vi "A2ii.vi"() -> ()   [LabVIEW 2020]
panel:
  out "Table":string[][](table)
  in  "stop":bool
  out "Sine":dynamicdata(graph)
  out "Mean":dbl
  in  "Enable":bool=TRUE
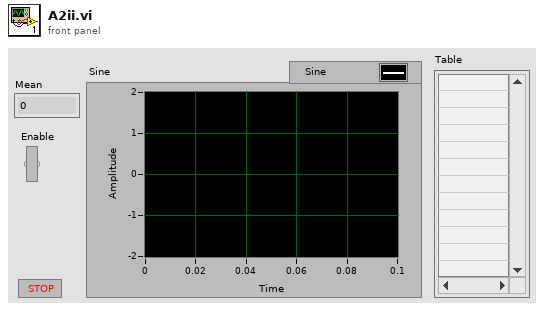
[diagram p1: front panel]
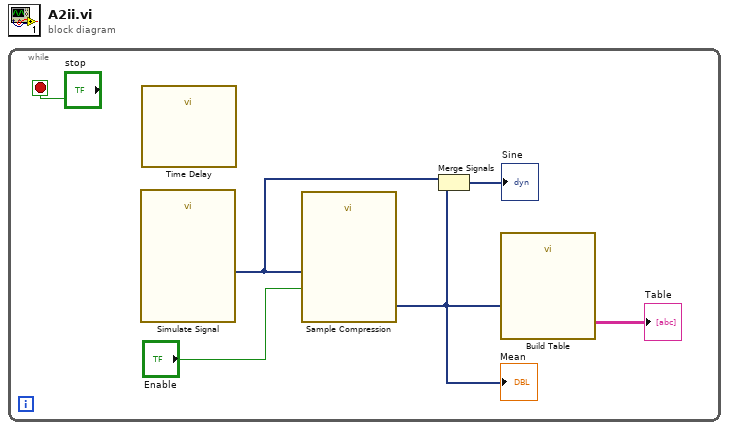
[diagram p0: block diagram]
diagram:
  n1 = while {
    stop <- "stop" stop-if-true
    n2 = call "Simulate Signal"() -> ("Sine"=w2:dynamicdata)  [unwired: 14 in, 1 out]
    n3 = call "Time Delay"() -> ()  [unwired: 11 in, 1 out]
    n4 = call "Sample Compression"("Enable"="Enable", "Signals"=w2) -> ("Mean"=w5:dynamicdata)  [unwired: 7 in, 2 out]
    "Mean" <- w5
    n5 = Merge Signals(w2, w5) -> (→"Sine":dynamicdata)
    n6 = call "Build Table"("Signals"=w5) -> ("Table"=→"Table":string[][])  [unwired: 4 in, 6 out]
  }
